vi "Define_Indicies_(101+Empty)_of_Affected_Tracks-1.vi"(4 "error IN":errorcluster, 5 "[IN] Subtracks":T2(array[cluster]), 6 "[IN] Indicies of sub\ntracks for transforma\ntion (resolving)":i32[](array[numeric]), 7 "[IN] Still connected\ntracks in group":T1) -> (0 "error OUT":errorcluster, 2 "[OUT] Indicies for Tr-\nack Reconstruction":i32[](array[numeric]))   [LabVIEW 2013]
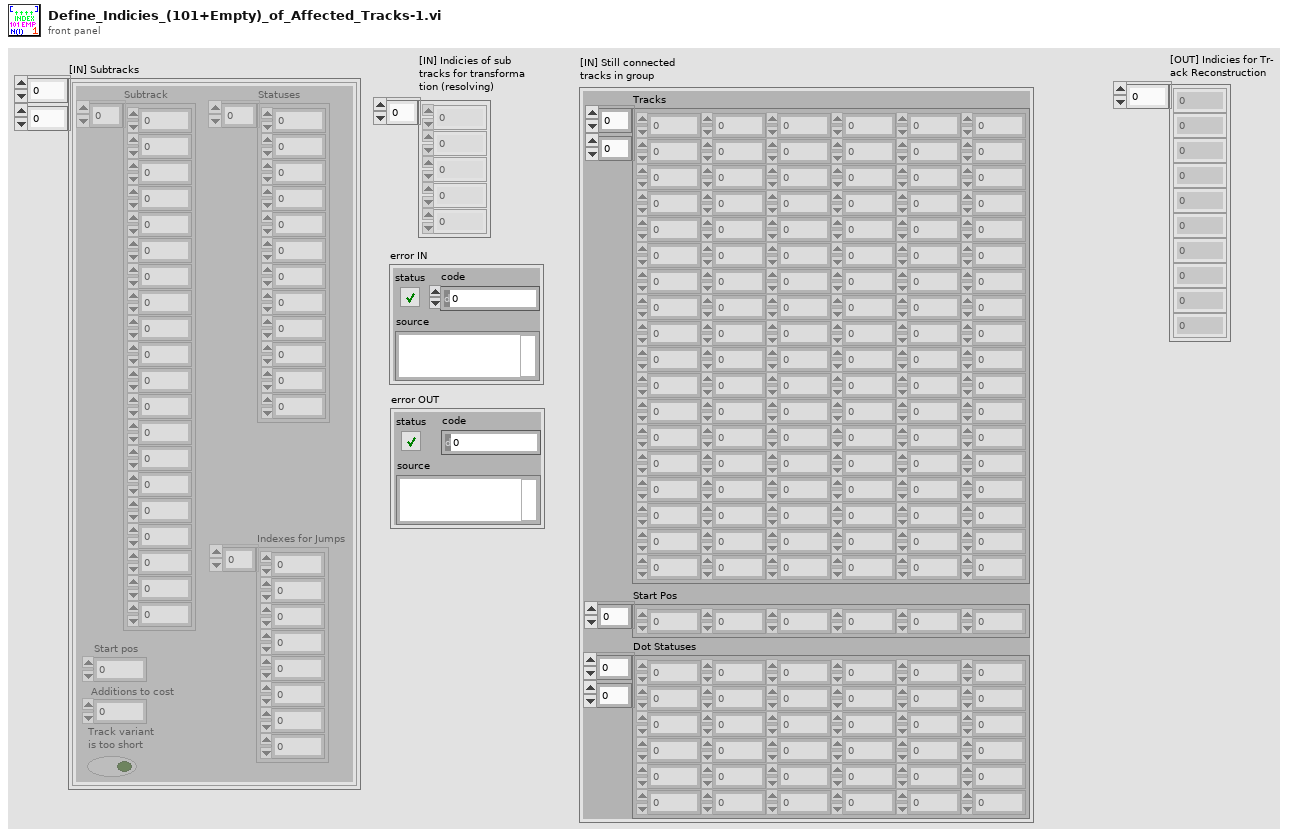
[diagram p1: front panel]
types:
  T1 = cluster{"Tracks":dbl[][], "Start Pos":i32[], "Dot Statuses":i16[][]}
  T2 = cluster{"Subtrack":dbl[], "Statuses":i16[], "Start pos":i32, "Additions to cost":i32, "Track variant \nis too short":bool, "Indexes for Jumps":i32[]}[][]
  T3 = cluster{"Subtrack":dbl[], "Statuses":i16[], "Start pos":i32, "Additions to cost":i32, "Track variant \nis too short":bool, "Indexes for Jumps":i32[]}
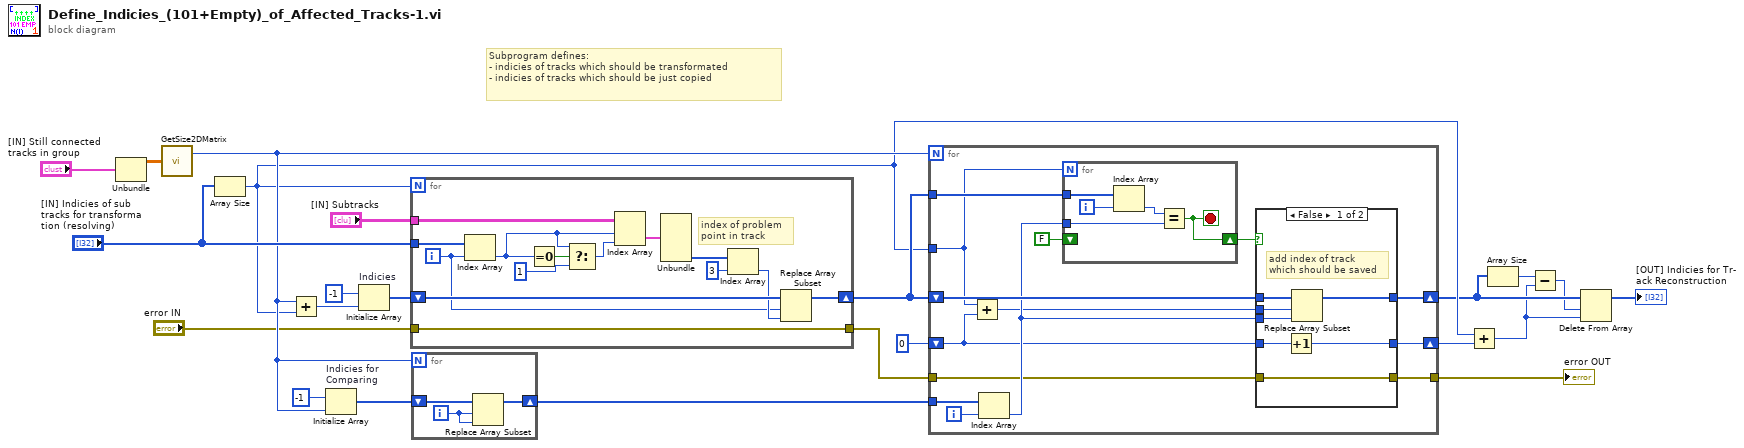
[diagram p0: block diagram]
diagram:
  # "Subprogram defines:\n- indicies of tracks which should be transformated\n- indicies of tracks which should be just copied"
  n1 = Unbundle("[IN] Still connected\ntracks in group") -> ("Tracks"=w20:dbl[][])  [unwired: 2 out]
  n2 = call "GetSize2DMatrix.vi"("Array IN (2D)"=w20) -> ("# Cols"=w13:i32)  [unwired: 1 out]
  n3 = Array Size(array="[IN] Indicies of sub\ntracks for transforma\ntion (resolving)") -> (size(s)=w10:i32)
  n4 = Add(x=w13, y=w10) -> (x+y=w19:i32)
  n5 = Initialize Array "Indicies for \nComparing"(-1 ("# Cols"), w13) -> (w15:i32[])
  n6 = Initialize Array "Indicies"(-1 ("# Cols"), w19) -> (w17:i32[])
  n7 = for {
    N: w10 -> [_]
    tunnel: "[IN] Subtracks" -> [w37]
    tunnel: "[IN] Indicies of sub\ntracks for transforma\ntion (resolving)" -> [w36]
    shift-right: [w29] -> w12
    shift-left: w17 -> [w32]
    tunnel: "error IN" -> [w28]
    tunnel: [w28] -> w2
    i -> [w30]
    # "index of problem \npoint in track"
    n8 = Index Array(array=w36, index=w30) -> (element=w24:i32)
    n9 = Equal To 0?(x=w24) -> (x = 0?=w27:bool)
    n10 = Select(t=w24, s=w27, f=1) -> (s? t:f=w25:i32)
    n11 = Index Array(array=w37, index (row)=w24, index (col)=w25) -> (element=w35:T3)
    n12 = Unbundle(w35) -> ("Indexes for Jumps"=w34:i32[])  [unwired: 5 out]
    n13 = Index Array(array=w34, index=3) -> (element=w31:i32)
    n14 = Replace Array Subset(array=w32, new element=w31, index=w30) -> (w29:i32[])
  }
  n15 = for {
    N: w13 -> [_]
    shift-right: [w38] -> w14
    shift-left: w15 -> [w40]
    i -> [w39]
    n16 = Replace Array Subset(array=w40, new element=w39, index=w39) -> (w38:i32[])
  }
  n17 = for {
    N: w13 -> [_]
    tunnel: w10 -> [w46]
    shift-right: [w48] -> w8
    shift-left: w12 -> [w49]
    tunnel: w14 -> [w54]
    tunnel: w12 -> [w52]
    shift-right: [w43] -> w9
    shift-left: 0 -> [w44]
    tunnel: w2 -> [w42]
    tunnel: [w41] -> w1
    i -> [w53]
    n18 = Add(x=w46, y=w44) -> (x+y=w45:i32)
    n19 = Index Array(array=w54, index=w53) -> (element=w47:i32)
    n20 = for {
      N: w46 -> [_]
      tunnel: w52 -> [w69]
      tunnel: w47 -> [w66]
      shift-right: [w65] -> w50
      shift-left: FALSE -> [_]
      i -> [w68]
      stop <- w65 stop-if-true
      n21 = Index Array(array=w69, index=w68) -> (element=w67:i32)
      n22 = Equal?(x=w67, y=w66) -> (x = y?=w65:bool)
    }
    n23 = case shown="False" w50 {
      tunnel: w49 -> [w61 w64]
      tunnel: [w58 w64] -> w48
      tunnel: w47 -> [w60 _]
      tunnel: w45 -> [w59 _]
      tunnel: w44 -> [w57 w63]
      tunnel: [w56 w63] -> w43
      tunnel: w42 -> [w55 w62]
      tunnel: [w55 w62] -> w41
      frame False {
        # "add index of track\nwhich should be saved"
        n24 = Increment(x=w57) -> (x+1=w56:i32)
        n25 = Replace Array Subset(array=w61, new element=w60, index=w59) -> (w58:i32[])
      }
      frame True {
      }
    }
  }
  "error OUT" <- w1
  n26 = Add(x=w10, y=w9) -> (x+y=w6:i32)
  n27 = Array Size(array=w8) -> (size(s)=w7:i32)
  n28 = Subtract(x=w7, y=w6) -> (x-y=w5:i32)
  n29 = Delete From Array(array=w8, length=w5, index=w6) -> (array with subset deleted=→"[OUT] Indicies for Tr-\nack Reconstruction":i32[])  [unwired: 1 out]
